vi "Valve_EPICS_Dev2.vi"() -> ()   [LabVIEW 2014]
uses:
  <userlib>/caLab/Private/Get_PV-1D.vi
  <userlib>/caLab/Private/Put_DBL-1D_PV-1D.vi
panel:
  out "ACT7":bool
  out "ACT6":bool
  out "ACT5":bool
  out "ACT4":bool
  out "ACT3":bool
  out "ACT2":bool
  out "ACT1":bool
  out "ACT0":bool
  in  "ENB7":bool
  in  "ENB6":bool
  in  "ENB5":bool
  in  "ENB4":bool
  in  "ENB3":bool
  in  "ENB2":bool
  in  "ENB1":bool
  in  "ENB0":bool
  out "initialized array":i16[](array[numeric])
  in  "stop":bool
  out "sum":i16
  out "0, 1":i16[](array[numeric])
  out "appended array":bool[](array[boolean])
  out "SCL_data":u32[](array[numeric]) caption="data"
  out "SOP_data":u32[](array[numeric]) caption="data"
  out "SCL7":bool
  out "SCL6":bool
  out "SCL5":bool
  out "SCL4":bool
  out "SCL3":bool
  out "SCL2":bool
  out "SCL1":bool
  out "SCL0":bool
  out "SOP7":bool
  out "SOP6":bool
  out "SOP5":bool
  out "SOP4":bool
  out "SOP3":bool
  out "SOP2":bool
  out "SOP1":bool
  out "SOP0":bool
  in  "OPEN7":bool
  in  "OPEN6":bool
  in  "OPEN5":bool
  in  "OPEN4":bool
  in  "OPEN3":bool
  in  "OPEN2":bool
  in  "OPEN1":bool
  in  "OPEN0":bool
  # "Valve control DEV4"
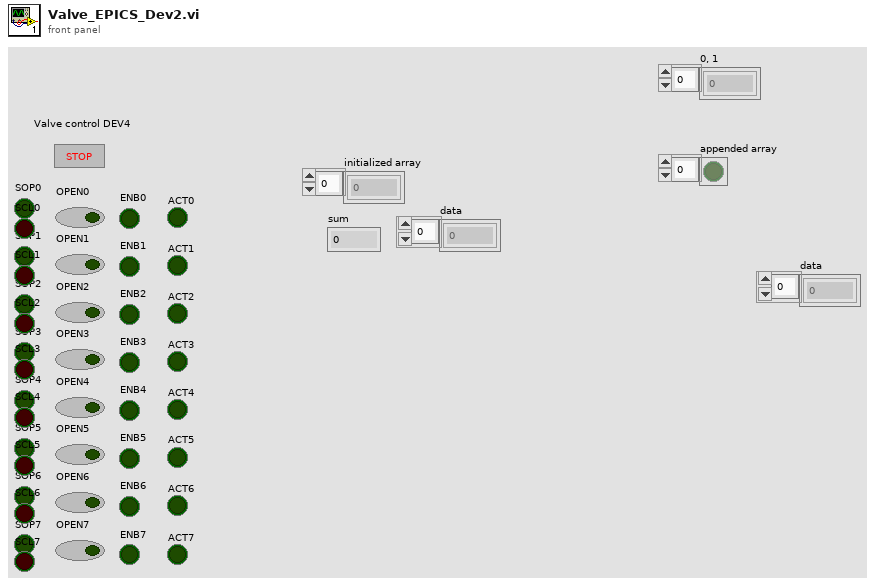
[diagram p1: front panel]
types:
  T1 = typedef "NI_Matrix.lvlib/RealMatrix.ctl" = dbl[][]
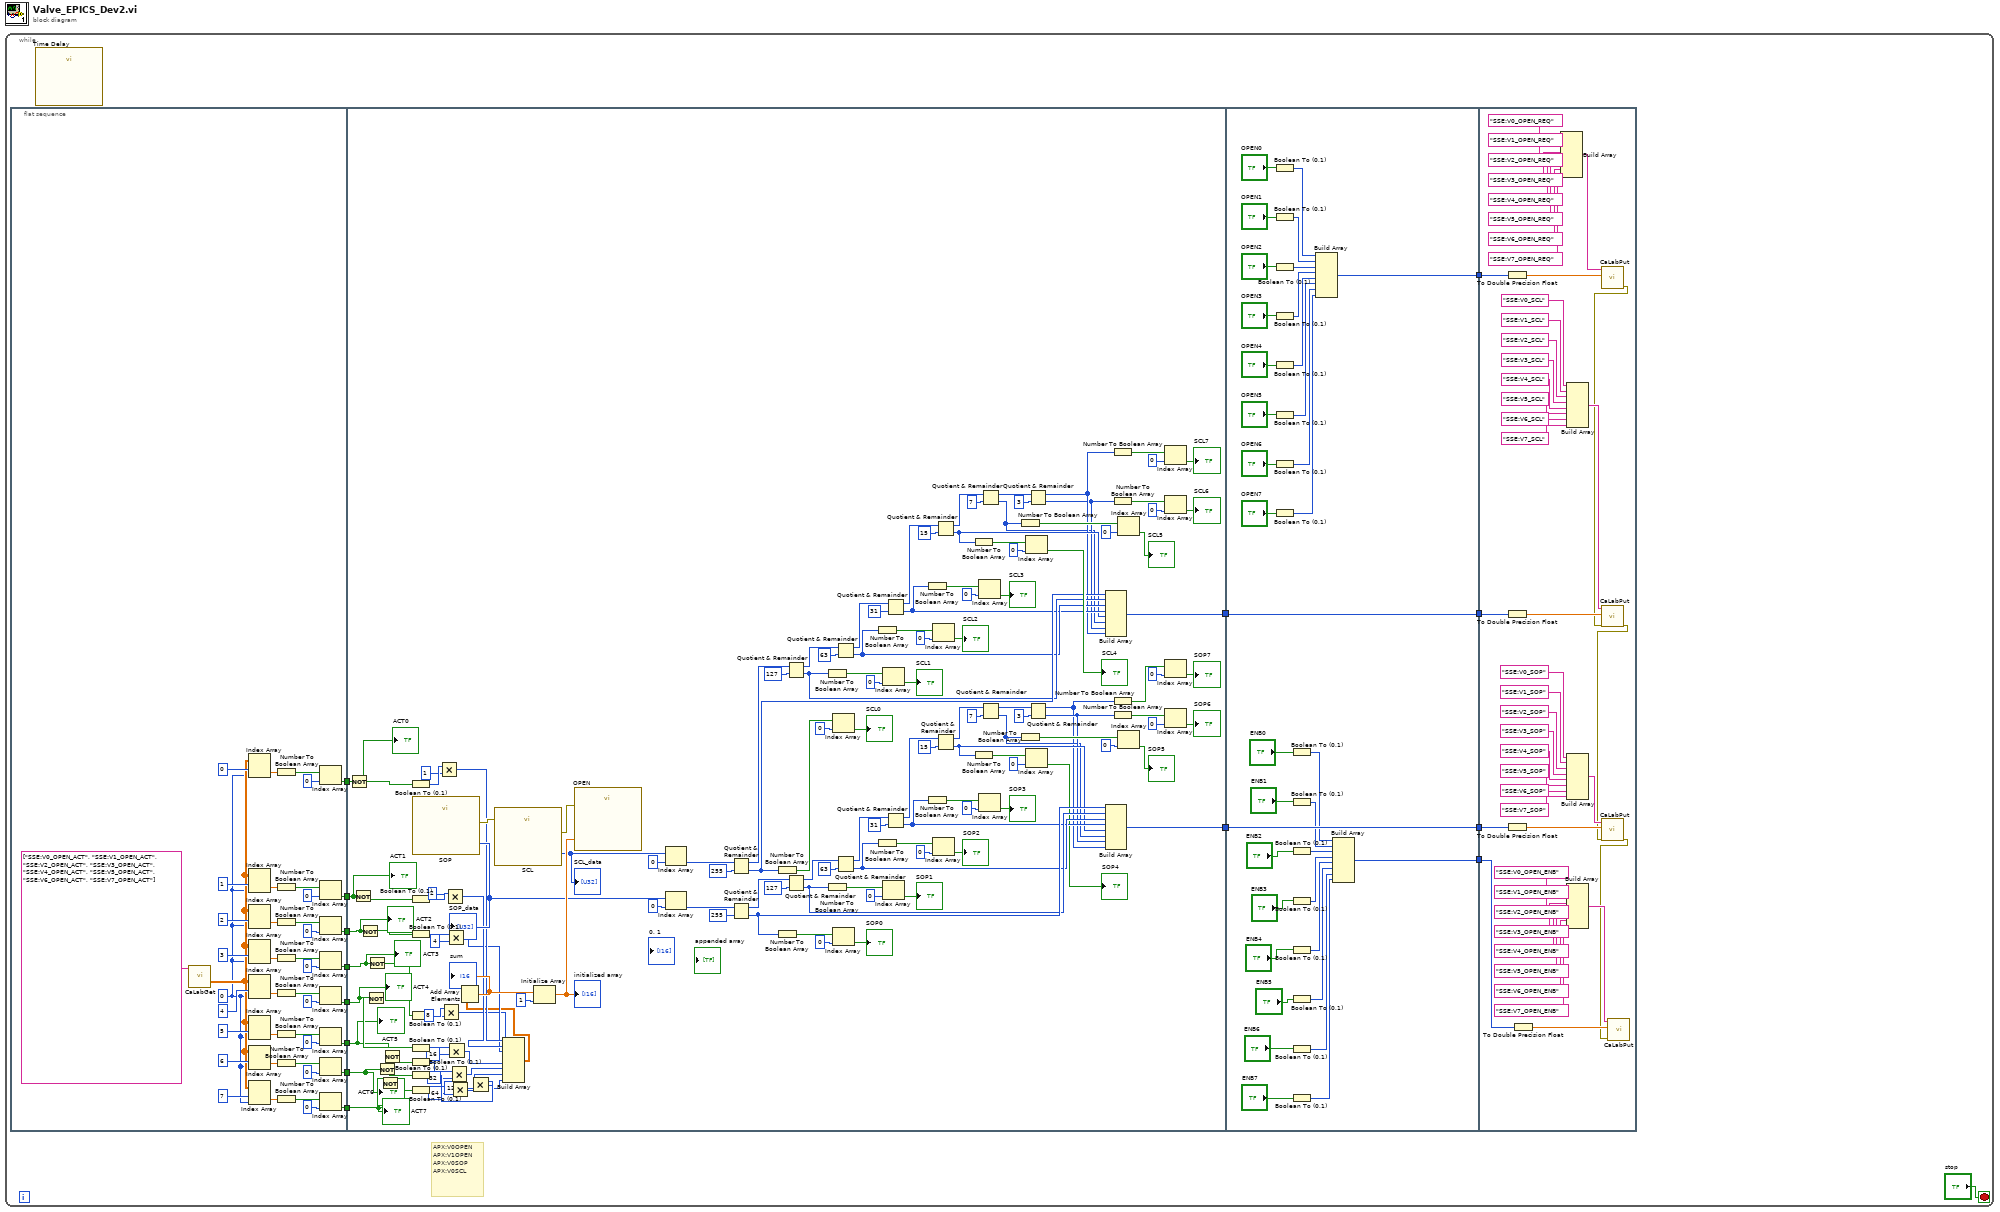
[diagram p0: block diagram]
diagram:
  n1 = while {
    stop <- "stop" stop-if-true
    # "APX:V0OPEN\nAPX:V1OPEN\nAPX:V0SOP\nAPX:V0SCL"
    n2 = flat-sequence {
      tunnel: [w23] -> w15
      tunnel: [w22] -> w14
      tunnel: [w21] -> w13
      tunnel: [w20] -> w12
      tunnel: [w19] -> w11
      tunnel: [w18] -> w10
      tunnel: [w17] -> w9
      tunnel: [w16] -> w8
      tunnel: w15 -> [w60]
      tunnel: w14 -> [w61]
      tunnel: w13 -> [w62]
      tunnel: w12 -> [w67]
      tunnel: w11 -> [w59]
      tunnel: w10 -> [w63]
      tunnel: w9 -> [w64]
      tunnel: w8 -> [w65]
      tunnel: [w149] -> w7
      tunnel: [w100] -> w3
      tunnel: w7 -> [w238]
      tunnel: [w238] -> w6
      tunnel: [w221] -> w5
      tunnel: w3 -> [w220]
      tunnel: [w220] -> w2
      tunnel: [w203] -> w1
      tunnel: w6 -> [w258]
      tunnel: w5 -> [w256]
      tunnel: w2 -> [w254]
      tunnel: w1 -> [w242]
      frame #0 {
        w48 = 0 ("index")
        n3 = call-poly "CaLabGet.vi"("PV Names"=string[] ["SSE:V0_OPEN_ACT", "SSE:V1_OPEN_ACT", "SSE:V2_OPEN_ACT", "SSE:V3_OPEN_ACT", "SSE:V4_OPEN_ACT", "SSE:V5_OPEN_ACT", "SSE:V6_OPEN_ACT", "SSE:V7_OPEN_ACT"]) -> ("Value Array (number)"=w49:dbl[][])  [unwired: 8 in, 6 out]
        n4 = Index Array(array=w49, index (row)=0 ("disabled index (row)"), index (col)=w48) -> (element=w28:dbl)
        n5 = Index Array(array=w49, index (row)=1, index (col)=w48) -> (element=w27:dbl)
        n6 = Index Array(array=w49, index (row)=2, index (col)=w48) -> (element=w31:dbl)
        n7 = Index Array(array=w49, index (row)=3 ("index"), index (col)=w48) -> (element=w30:dbl)
        n8 = Index Array(array=w49, index (row)=4, index (col)=w48) -> (element=w29:dbl)
        n9 = Index Array(array=w49, index (row)=5, index (col)=w48) -> (element=w26:dbl)
        n10 = Index Array(array=w49, index (row)=6, index (col)=w48) -> (element=w25:dbl)
        n11 = Index Array(array=w49, index (row)=7, index (col)=w48) -> (element=w24:dbl)
        n12 = Number To Boolean Array(number=w28) -> (Boolean array=w41:bool[])
        n13 = Number To Boolean Array(number=w27) -> (Boolean array=w39:bool[])
        n14 = Number To Boolean Array(number=w31) -> (Boolean array=w47:bool[])
        n15 = Number To Boolean Array(number=w30) -> (Boolean array=w45:bool[])
        n16 = Number To Boolean Array(number=w29) -> (Boolean array=w43:bool[])
        n17 = Number To Boolean Array(number=w26) -> (Boolean array=w37:bool[])
        n18 = Number To Boolean Array(number=w25) -> (Boolean array=w35:bool[])
        n19 = Number To Boolean Array(number=w24) -> (Boolean array=w33:bool[])
        n20 = Index Array(array=w41, index=0) -> (element=w20:bool)
        n21 = Index Array(array=w39, index=0) -> (element=w19:bool)
        n22 = Index Array(array=w47, index=0) -> (element=w23:bool)
        n23 = Index Array(array=w45, index=0) -> (element=w22:bool)
        n24 = Index Array(array=w43, index=0) -> (element=w21:bool)
        n25 = Index Array(array=w37, index=0) -> (element=w18:bool)
        n26 = Index Array(array=w35, index=0) -> (element=w17:bool)
        n27 = Index Array(array=w33, index=0) -> (element=w16:bool)
      }
      frame #1 {
        n28 = Not(x=w67) -> (.not. x?=w66:bool)
        n29 = Not(x=w59) -> (.not. x?=w91:bool)
        n30 = Not(x=w60) -> (.not. x?=w90:bool)
        n31 = Not(x=w62) -> (.not. x?=w88:bool)
        n32 = Not(x=w61) -> (.not. x?=w89:bool)
        n33 = Not(x=w64) -> (.not. x?=w86:bool)
        n34 = Not(x=w65) -> (.not. x?=w85:bool)
        n35 = Not(x=w63) -> (.not. x?=w87:bool)
        n36 = Boolean To (0,1)(Boolean=w66) -> (0, 1=w99:i16)
        n37 = Boolean To (0,1)(Boolean=w91) -> (0, 1=w98:i16)
        n38 = Boolean To (0,1)(Boolean=w90) -> (0, 1=w97:i16)
        n39 = Boolean To (0,1)(Boolean=w89) -> (0, 1=w96:i16)
        n40 = Boolean To (0,1)(Boolean=w88) -> (0, 1=w95:i16)
        n41 = Boolean To (0,1)(Boolean=w87) -> (0, 1=w94:i16)
        n42 = Boolean To (0,1)(Boolean=w86) -> (0, 1=w93:i16)
        n43 = Boolean To (0,1)(Boolean=w85) -> (0, 1=w92:i16)
        n44 = call "SOP"() -> ("data"=w112:u32[], "error out"=w177:errorcluster)  [unwired: 17 in, 1 out]
        "SOP_data" <- w112
        n45 = Multiply(x=w99, y=i16 1) -> (x*y=w76:i16)
        n46 = Multiply(x=w96, y=i16 8) -> (x*y=w73:i16)
        n47 = Multiply(x=w98, y=i16 2) -> (x*y=w75:i16)
        n48 = Multiply(x=w97, y=i16 4) -> (x*y=w74:i16)
        n49 = Multiply(x=w95, y=i16 16) -> (x*y=w72:i16)
        n50 = Multiply(x=w94, y=i16 32) -> (x*y=w71:i16)
        n51 = Multiply(x=w93, y=i16 64) -> (x*y=w70:i16)
        n52 = Multiply(x=w92, y=i16 128) -> (x*y=w69:i16)
        n53 = call "SCL"("error in"=w177) -> ("data"=w172:u32[], "error out"=w176:errorcluster)  [unwired: 16 in, 1 out]
        "SCL_data" <- w172
        n54 = Build Array(w76, w75, w74, w73, w72, w71, w70, w69) -> (w68:T1)
        n55 = Add Array Elements(numeric array=w68) -> (sum=w174:dbl)
        "sum" <- w174
        n56 = Initialize Array(w174, 1 ("dimension size")) -> (w173:dbl[])
        "initialized array" <- w173
        n57 = call "OPEN"("data"=w173, "error in"=w176) -> ()  [unwired: 16 in, 2 out]
        n58 = Index Array(array=w172, index=0) -> (element=w171:u32)
        n59 = Index Array(array=w112, index=0) -> (element=w111:u32)
        n60 = Quotient & Remainder(x=w171, y=u32 255) -> (x-y*floor(x/y)=w169:u32, floor(x/y)=w157:u32)
        n61 = Quotient & Remainder(x=w111, y=u32 255) -> (x-y*floor(x/y)=w132:u32, floor(x/y)=w120:u32)
        n62 = Number To Boolean Array(number=w157) -> (Boolean array=w201:bool[])
        n63 = Number To Boolean Array(number=w120) -> (Boolean array=w148:bool[])
        n64 = Quotient & Remainder(x=w169, y=u32 127) -> (x-y*floor(x/y)=w164:u32, floor(x/y)=w156:u32)
        n65 = Quotient & Remainder(x=w132, y=u32 127) -> (x-y*floor(x/y)=w127:u32, floor(x/y)=w119:u32)
        n66 = Number To Boolean Array(number=w156) -> (Boolean array=w199:bool[])
        n67 = Number To Boolean Array(number=w119) -> (Boolean array=w146:bool[])
        n68 = Index Array(array=w201, index=0) -> (element=→"SCL0":bool)
        n69 = Index Array(array=w148, index=0) -> (element=→"SOP0":bool)
        n70 = Quotient & Remainder(x=w164, y=u32 63) -> (x-y*floor(x/y)=w163:u32, floor(x/y)=w155:u32)
        n71 = Quotient & Remainder(x=w127, y=u32 63) -> (x-y*floor(x/y)=w126:u32, floor(x/y)=w118:u32)
        n72 = Number To Boolean Array(number=w155) -> (Boolean array=w197:bool[])
        n73 = Number To Boolean Array(number=w118) -> (Boolean array=w144:bool[])
        n74 = Index Array(array=w199, index=0) -> (element=→"SCL1":bool)
        n75 = Index Array(array=w146, index=0) -> (element=→"SOP1":bool)
        n76 = Quotient & Remainder(x=w163, y=u32 31) -> (x-y*floor(x/y)=w162:u32, floor(x/y)=w154:u32)
        n77 = Quotient & Remainder(x=w126, y=u32 31) -> (x-y*floor(x/y)=w125:u32, floor(x/y)=w117:u32)
        n78 = Number To Boolean Array(number=w154) -> (Boolean array=w195:bool[])
        n79 = Number To Boolean Array(number=w117) -> (Boolean array=w142:bool[])
        n80 = Index Array(array=w197, index=0) -> (element=→"SCL2":bool)
        n81 = Index Array(array=w144, index=0) -> (element=→"SOP2":bool)
        n82 = Quotient & Remainder(x=w162, y=u32 15) -> (x-y*floor(x/y)=w159:u32, floor(x/y)=w153:u32)
        n83 = Quotient & Remainder(x=w125, y=u32 15) -> (x-y*floor(x/y)=w122:u32, floor(x/y)=w116:u32)
        n84 = Number To Boolean Array(number=w153) -> (Boolean array=w193:bool[])
        n85 = Number To Boolean Array(number=w116) -> (Boolean array=w140:bool[])
        n86 = Index Array(array=w195, index=0) -> (element=→"SCL3":bool)
        n87 = Index Array(array=w142, index=0) -> (element=→"SOP3":bool)
        n88 = Quotient & Remainder(x=w159, y=u32 7) -> (x-y*floor(x/y)=w158:u32, floor(x/y)=w150:u32)
        n89 = Quotient & Remainder(x=w122, y=u32 7) -> (x-y*floor(x/y)=w121:u32, floor(x/y)=w114:u32)
        n90 = Number To Boolean Array(number=w150) -> (Boolean array=w191:bool[])
        n91 = Number To Boolean Array(number=w114) -> (Boolean array=w138:bool[])
        n92 = Index Array(array=w193, index=0) -> (element=→"SCL4":bool)
        n93 = Index Array(array=w140, index=0) -> (element=→"SOP4":bool)
        n94 = Quotient & Remainder(x=w158, y=u32 3) -> (x-y*floor(x/y)=w152:u32, floor(x/y)=w151:u32)
        n95 = Quotient & Remainder(x=w121, y=u32 3) -> (x-y*floor(x/y)=w104:u32, floor(x/y)=w115:u32)
        n96 = Build Array(w157, w156, w155, w154, w153, w150, w151, w152) -> (w149:u32[])
        n97 = Build Array(w120, w119, w118, w117, w116, w114, w115, w104) -> (w100:u32[])
        n98 = Number To Boolean Array(number=w152) -> (Boolean array=w187:bool[])
        n99 = Number To Boolean Array(number=w151) -> (Boolean array=w189:bool[])
        n100 = Number To Boolean Array(number=w104) -> (Boolean array=w103:bool[])
        n101 = Number To Boolean Array(number=w115) -> (Boolean array=w136:bool[])
        n102 = Index Array(array=w191, index=0) -> (element=→"SCL5":bool)
        n103 = Index Array(array=w138, index=0) -> (element=→"SOP5":bool)
        n104 = Index Array(array=w187, index=0) -> (element=→"SCL7":bool)
        n105 = Index Array(array=w189, index=0) -> (element=→"SCL6":bool)
        n106 = Index Array(array=w103, index=0) -> (element=→"SOP7":bool)
        n107 = Index Array(array=w136, index=0) -> (element=→"SOP6":bool)
        "ACT0" <- w67
        "ACT7" <- w65
        "ACT6" <- w64
        "ACT5" <- w63
        "ACT4" <- w62
        "ACT3" <- w61
        "ACT2" <- w60
        "ACT1" <- w59
      }
      frame #2 {
        n108 = Boolean To (0,1)(Boolean="OPEN0") -> (0, 1=w237:i16)
        n109 = Boolean To (0,1)(Boolean="OPEN1") -> (0, 1=w236:i16)
        n110 = Boolean To (0,1)(Boolean="OPEN2") -> (0, 1=w235:i16)
        n111 = Boolean To (0,1)(Boolean="OPEN3") -> (0, 1=w234:i16)
        n112 = Boolean To (0,1)(Boolean="OPEN4") -> (0, 1=w233:i16)
        n113 = Boolean To (0,1)(Boolean="OPEN5") -> (0, 1=w232:i16)
        n114 = Boolean To (0,1)(Boolean="OPEN6") -> (0, 1=w231:i16)
        n115 = Boolean To (0,1)(Boolean="OPEN7") -> (0, 1=w230:i16)
        n116 = Boolean To (0,1)(Boolean="ENB0") -> (0, 1=w219:i16)
        n117 = Boolean To (0,1)(Boolean="ENB1") -> (0, 1=w218:i16)
        n118 = Boolean To (0,1)(Boolean="ENB2") -> (0, 1=w217:i16)
        n119 = Boolean To (0,1)(Boolean="ENB3") -> (0, 1=w216:i16)
        n120 = Boolean To (0,1)(Boolean="ENB4") -> (0, 1=w215:i16)
        n121 = Boolean To (0,1)(Boolean="ENB5") -> (0, 1=w214:i16)
        n122 = Boolean To (0,1)(Boolean="ENB6") -> (0, 1=w213:i16)
        n123 = Boolean To (0,1)(Boolean="ENB7") -> (0, 1=w212:i16)
        n124 = Build Array(w237, w236, w235, w234, w233, w232, w231, w230) -> (w221:i16[])
        n125 = Build Array(w219, w218, w217, w216, w215, w214, w213, w212) -> (w203:i16[])
      }
      frame #3 {
        n126 = To Double Precision Float(number=w256) -> (double precision float=w255:dbl[])
        n127 = To Double Precision Float(number=w258) -> (double precision float=w257:dbl[])
        n128 = To Double Precision Float(number=w254) -> (double precision float=w259:dbl[])
        n129 = To Double Precision Float(number=w242) -> (double precision float=w244:dbl[])
        n130 = Build Array("SSE:V0_OPEN_REQ", "SSE:V1_OPEN_REQ", "SSE:V2_OPEN_REQ", "SSE:V3_OPEN_REQ", "SSE:V4_OPEN_REQ", "SSE:V5_OPEN_REQ", "SSE:V6_OPEN_REQ", "SSE:V7_OPEN_REQ") -> (w261:string[])
        n131 = Build Array("SSE:V0_SCL", "SSE:V1_SCL", "SSE:V2_SCL", "SSE:V3_SCL", "SSE:V4_SCL", "SSE:V5_SCL", "SSE:V6_SCL", "SSE:V7_SCL") -> (w260:string[])
        n132 = Build Array("SSE:V0_SOP", "SSE:V1_SOP", "SSE:V2_SOP", "SSE:V3_SOP", "SSE:V4_SOP", "SSE:V5_SOP", "SSE:V6_SOP", "SSE:V7_SOP") -> (w253:string[])
        n133 = Build Array("SSE:V0_OPEN_ENB", "SSE:V1_OPEN_ENB", "SSE:V2_OPEN_ENB", "SSE:V3_OPEN_ENB", "SSE:V4_OPEN_ENB", "SSE:V5_OPEN_ENB", "SSE:V6_OPEN_ENB", "SSE:V7_OPEN_ENB") -> (w243:string[])
        n134 = call-poly <userlib>:"CaLabPut.vi"("Values"=w255, "PV Names"=w261) -> ("Error out"=w239:errorcluster)  [unwired: 6 in, 3 out]
        n135 = call-poly <userlib>:"CaLabPut.vi"("Error in (no error)"=w239, "Values"=w257, "PV Names"=w260) -> ("Error out"=w240:errorcluster)  [unwired: 5 in, 3 out]
        n136 = call-poly <userlib>:"CaLabPut.vi"("Error in (no error)"=w240, "Values"=w259, "PV Names"=w253) -> ("Error out"=w241:errorcluster)  [unwired: 5 in, 3 out]
        n137 = call-poly <userlib>:"CaLabPut.vi"("Error in (no error)"=w241, "Values"=w244, "PV Names"=w243) -> ()  [unwired: 5 in, 4 out]
      }
    }
    n138 = call "Time Delay"() -> ()  [unwired: 11 in, 1 out]
  }
